vi "FPGA_AIReadAccumulatorOutput.vi"(8 "error in (no error)":errorcluster, 10 "Channel":T1=enum."AI 1", 11 "AI Reference":T2) -> (0 "error out":errorcluster, 1 "Count":u32, 2 "Value":i64, 3 "AI Reference":T2)   [LabVIEW 2017]
uses:
  <vilib>/Rock Robotics/SystemInterfaces/AI/FPGA_AIDevRef.ctl
  <vilib>/Rock Robotics/SystemInterfaces/AI/FPGA_AIChannel.ctl
  <vilib>/Rock Robotics/SystemInterfaces/System/FPGA_SystemFPGA Ref Global.vi
  <vilib>/Utility/error.llb/Error Cluster From Error Code.vi
  <vilib>/rvi/errors/niLvFpgaAdjustHostInterfaceError.vi
  <vilib>/rvi/interface/nirviReadWriteControl/nirviReadWriteControl.xnode
  <vilib>/Rock Robotics/SystemInterfaces/System/FPGA_SystemFRC FPGA Ref.ctl
  <vilib>/rvi/interface/Simulation/niFpgaSimulationCallBeginRW.vi
  NiFpgaLv.dll
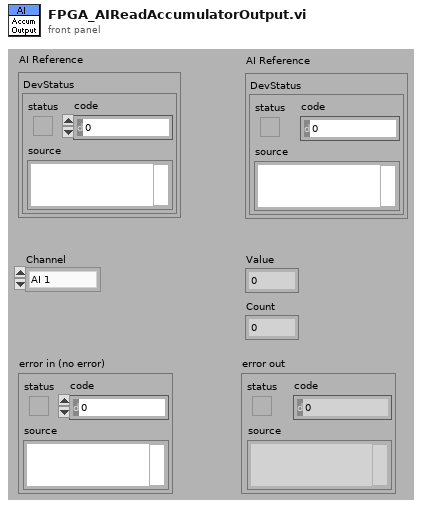
[diagram p1: front panel]
types:
  T1 = typedef "FPGA_AIChannel.ctl" = enum8{"AI 0", "AI 1", "AI 2", "AI 3", "AI MXP 0", "AI MXP 1", "AI MXP 2", "AI MXP 3", "Invalid"}
  T2 = typedef "FPGA_AIDevRef.ctl" = cluster{"DevStatus":errorcluster}
  T3 = typedef "FPGA_SystemFRC FPGA Ref.ctl" = refnum<k20>
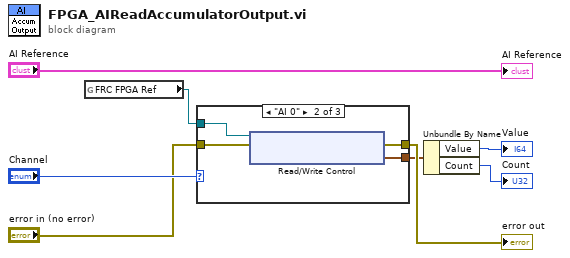
[diagram p0: block diagram]
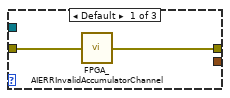
[diagram p2: hidden frame]
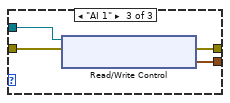
[diagram p3: hidden frame]
diagram:
  n1 = global read "FPGA_SystemFPGA Ref Global.vi" "FRC FPGA Ref"() -> (w2:T3)
  n2 = case shown="\"AI 0\"" "Channel" {
    tunnel: "error in (no error)" -> [w10 w11 w16]
    tunnel: [w9 w14 w18] -> w6
    tunnel: [_ w13 w17] -> w3
    tunnel: w2 -> [_ w12 w15]
    frame Default {
      n3 = call <vilib>:"FPGA_AIERRInvalidAccumulatorChannel.vi"("error in (no error)"=w10) -> ("error out"=w9:errorcluster)
    }
    frame "AI 0" {
      n4 = xnode "Read/Write Control"("FPGA VI Reference In"=w12, "error in"=w11) -> ("error out"=w14:errorcluster, "Accumulator0.Output"=w13:cluster{"Value":i64, "Count":u32})  [unwired: 1 out]
    }
    frame "AI 1" {
      n5 = xnode "Read/Write Control"("FPGA VI Reference In"=w15, "error in"=w16) -> ("error out"=w18:errorcluster, "Accumulator1.Output"=w17:cluster{"Value":i64, "Count":u32})  [unwired: 1 out]
    }
  }
  "error out" <- w6
  n6 = Unbundle By Name(w3) -> ("Value"=→"Value":i64, "Count"=→"Count":u32)
  "AI Reference" <- "AI Reference"
